vi "NN_Draw_Rectangle.vi"(4 "Clear Overlays?":bool=TRUE, 5 "font_size":sgl=20.0, 6 "Labels":string[](array[string])=["aeroplane", "bicycle", "bird", "boat", "bottle", "bus", "car", "cat", "chair", "cow", "diningtable", "dog", "horse", "motorbike", "person", "pottedplant", "sheep", "sofa", "train", "tvmonitor"], 7 "Border_Width":u32=4, 8 "error in (no error)":errorcluster, 9 "Colors":u32[](array[colorbox])=[6618880, 15679744, 6684927, 1638655, 13311, 33023, 52479, 65509, 65433, 65356, 65280, 5111552, 10092288, 15138560, 16763904, 16744192, 16724736, 16711680, 16711680, 16711680], 10 "Draw_Boxes":T1[](array[typedef]) {"BBox"."x" format="%#_4p"; "BBox"."y" format="%#_4p"; "BBox"."w" format="%#_4p"; "BBox"."h" format="%#_4p"}, 11 "Img in":T3=refnum) -> (0 "error out":errorcluster, 3 "Img out":T3)   [LabVIEW 2020]
doc: "Draws bounding box regtangles around objects on the image based on BBox input information ."
uses:
  <vilib>/vision/Image Controls.llb/IMAQ Image.ctl
  <vilib>/Ngene/Deep Learning Toolkit/Toolkit/NN_Data/API/Data/Detection_Types/NN_BBox_Detection.ctl
  <vilib>/Ngene/Deep Learning Toolkit/Toolkit/NN_Data/API/Data/Detection_Types/NN_BBox.ctl
  <vilib>/Ngene/Deep Learning Toolkit/Toolkit/NN_Data/API/NN_Dims(C,H,W).ctl
  <vilib>/Ngene/Deep Learning Toolkit/Toolkit/Deep_Learning_Toolkit_by_Ngene.lvlib
panel:
  out "Exec_Time(s)":dbl=0.000148600014654221
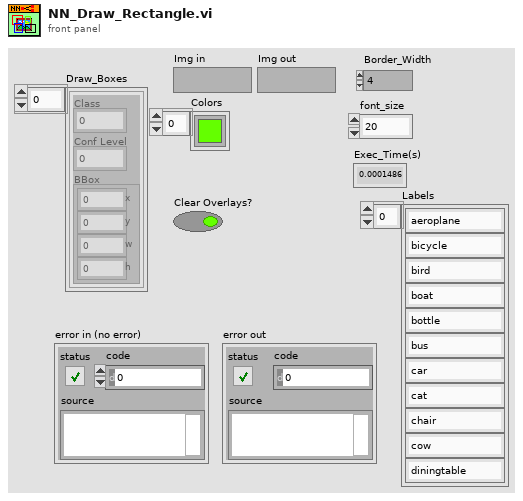
[diagram p1: front panel]
types:
  T1 = typedef "Deep_Learning_Toolkit_by_Ngene.lvlib/NN_BBox_Detection.ctl" = cluster{"Class":i32, "Conf Level":sgl, "BBox":T2}
  T2 = typedef "Deep_Learning_Toolkit_by_Ngene.lvlib/NN_BBox.ctl" = cluster{"x":sgl, "y":sgl, "w":sgl, "h":sgl}
  T3 = typedef "IMAQ Image.ctl" = refnum<image>
  T4 = typedef "Deep_Learning_Toolkit_by_Ngene.lvlib/NN_Dims(C,H,W).ctl" = cluster{"C":i32, "H":i32, "W":i32}
  T5 = cluster{"Desired Font (Application)":enum16{"User-specified Font", "Application Font", "System Font", "Dialog Font"}, "[User-specified Font]":cluster{"Font Name":string, "Size":i16, "Strikeout?":bool, "Italic?":bool, "Underline?":bool, "Outline?":bool, "Shadow?":bool, "Bold?":bool, "Rotation Angle":dbl}, "Horizontal Alignment":i16, "Vertical Alignment":i16}
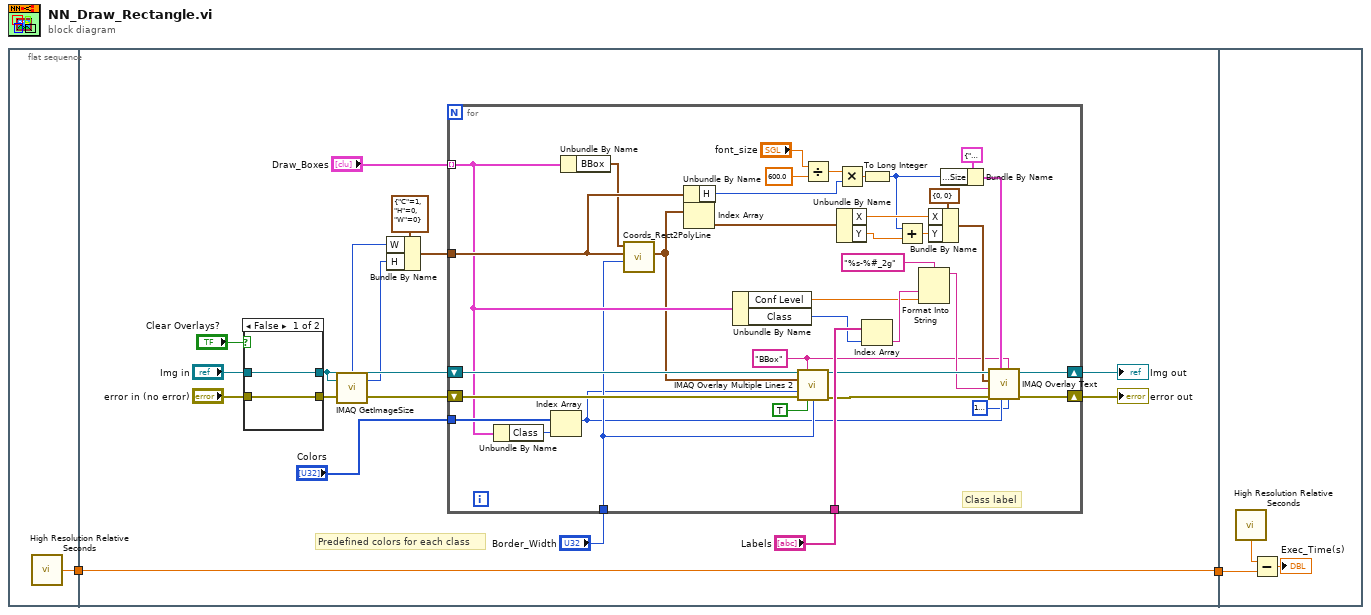
[diagram p0: block diagram]
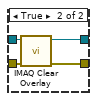
[diagram p2: hidden frame]
diagram:
  n1 = flat-sequence {
    tunnel: [w3] -> w2
    tunnel: w2 -> [w10]
    tunnel: [w10] -> w1
    tunnel: w1 -> [w66]
    frame #0 {
      n2 = call <vilib>:"High Resolution Relative Seconds.vi"() -> ("relative seconds"=w3:dbl)
    }
    frame #1 {
      # "Predefined colors for each class"
      n3 = case shown="False" "Clear Overlays?" {
        tunnel: "Img in" -> [w22 w26]
        tunnel: [w22 w25] -> w13
        tunnel: "error in (no error)" -> [w21 w24]
        tunnel: [w21 w23] -> w5
        frame False {
        }
        frame True {
          n4 = call "IMAQ Clear Overlay"("error in (no error)"=w24, "Image"=w26) -> ("error out"=w23:errorcluster, "Image Out"=w25:T3)  [unwired: 8 in]
        }
      }
      n5 = call "IMAQ GetImageSize"("Image"=w13, "error in (no error)"=w5) -> ("Y Resolution"=w11:i32, "X Resolution"=w12:i32, "error out"=w14:errorcluster)  [unwired: 2 in]
      n6 = Bundle By Name(cluster=T4 {"C"=1, "H"=0, "W"=0} ("In_Dims"), "W"=w12, "H"=w11) -> (w15:T4)
      n7 = for {
        tunnel: "Colors" -> [w63]
        shift-right: [w62] -> w20
        shift-left: w14 -> [w59]
        shift-right: [w61] -> w19
        shift-left: w13 -> [w58]
        tunnel: w15 -> [w60]
        tunnel: "Draw_Boxes" -> [w57] mode=indexing
        tunnel: "Border_Width" -> [w55]
        tunnel: "Labels" -> [w54]
        w39 = "BBox" ("Group")
        # "Class label"
        n8 = Unbundle By Name(w57) -> ("Class"=w56:i32)
        n9 = Index Array(array=w63, index=w56) -> (element=w28:u32)
        n10 = Unbundle By Name(w57) -> ("BBox"=w40:T2)
        n11 = call <vilib>:"Coords_Rect2PolyLine.vi"("Border_Width"=w55, "In_Dims"=w60, "BBox"=w40) -> ("PolyLine"=w33:cluster{"X":dbl, "Y":dbl}[])  [unwired: 8 in]
        n12 = Unbundle By Name(w60) -> ("H"=w34:i32)
        n13 = Index Array(array=w33) -> (element=w32:cluster{"X":dbl, "Y":dbl})  [unwired: 1 in]
        n14 = Unbundle By Name(w57) -> ("Conf Level"=w29:sgl, "Class"=w31:i32)
        n15 = call "IMAQ Overlay Multiple Lines 2"("Image"=w58, "Group"=w39, "Line End Points"=w33, "Color"=w28, "error in (no error)"=w59, "Maintain Width?"=TRUE, "Width"=w55) -> ("Image Out"=w53:T3, "error out"=w52:errorcluster)  [unwired: 7 in]
        n16 = Divide(x="font_size", y=sgl 600.0) -> (x/y=w42:sgl)
        n17 = Multiply(x=w42, y=w34) -> (x*y=w43:sgl)
        n18 = Unbundle By Name(w32) -> ("X"=w37:dbl, "Y"=w36:dbl)
        n19 = To Long Integer(number=w43) -> (32bit integer=w35:i32)
        n20 = Index Array(array=w54, index=w31) -> (element=w30:string)
        n21 = Add(x=w35, y=w36) -> (x+y=w49:dbl)
        n22 = Format Into String(format string="%s-%#_2g", w30, w29) -> (resulting string=w47:string)  [unwired: 2 in, 1 out]
        n23 = Bundle By Name(cluster=cluster{"X":i32, "Y":i32} {"X"=0, "Y"=0} ("Origin"), "X"=w37, "Y"=w49) -> (w50:cluster{"X":i32, "Y":i32})
        n24 = Bundle By Name(cluster=T5 {"Desired Font (Application)"=enum."User-specified Font", "[User-specified Font]"={"Font Name"="", "Size"=18, "Strikeout?"=FALSE, "Italic?"=FALSE, "Underline?"=FALSE, "Outline?"=FALSE, "Shadow?"=FALSE, "Bold?"=TRUE, "Rotation Angle"=0.0}, "Horizontal Alignment"=0, "Vertical Alignment"=0} ("Font, Size & Style"), "[User-specified Font].Size"=w35) -> (w45:T5)
        n25 = call "IMAQ Overlay Text"("BG Color (Transparent)"=u32 16777216, "Group"=w39, "Text Color (black)"=w28, "Font, Size & Style"=w45, "error in (no error)"=w52, "String"=w47, "Origin"=w50, "Image"=w53) -> ("error out"=w62:errorcluster, "Image Out"=w61:T3)  [unwired: 2 in]
      }
      "error out" <- w20
      "Img out" <- w19
    }
    frame #2 {
      n26 = call <vilib>:"High Resolution Relative Seconds.vi"() -> ("relative seconds"=w65:dbl)
      n27 = Subtract(x=w65, y=w66) -> (x-y=→"Exec_Time(s)":dbl)
    }
  }
